vi "Default Instrument Setup.vi"(8 "error in (no error)":errorcluster, 11 "VISA resource name":refnum<visa-resource-name>) -> (0 "error out":errorcluster, 3 "VISA resource name out":refnum<visa-resource-name>)   [LabVIEW 2021, in "Keithley 24XX.lvlib"]
doc: "This Utility VI sends a default command string to the instrument whenever a new VISA session is opened, or the instrument is reset. Use this VI as a subVI for the Initialize and Reset VIs. Altering this VI could cause these two VIs to operate incorrectly."
uses:
  <instrlib>/Keithley 24XX/Keithley 24XX.lvlib
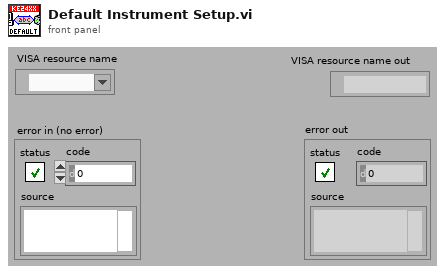
[diagram p1: front panel]
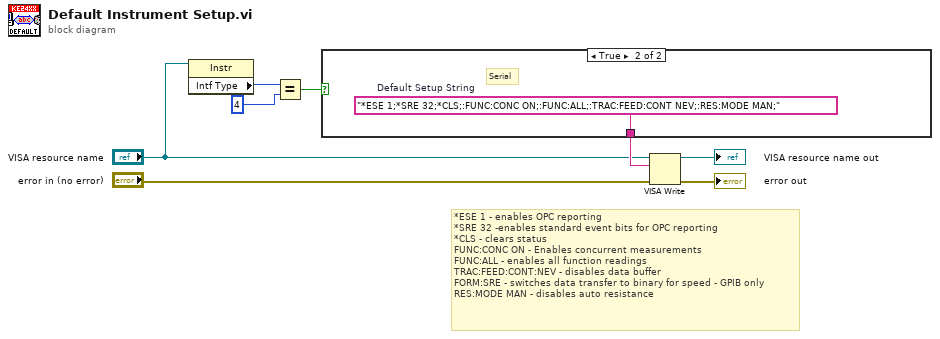
[diagram p0: block diagram]
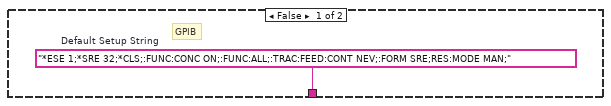
[diagram p2: hidden frame]
diagram:
  # "*ESE 1 - enables OPC reporting\n*SRE 32 -enables standard event bits for OPC reporting\n*CLS - clears status\nFUNC:CONC ON - Enables concurrent measurements\nFUNC:ALL - enables all function readings\nTRAC:FEED:CONT:NEV - disables data buffer\nFORM:SRE - switches data transfer to binary for speed - GPIB only\nRES:MODE MAN - disables auto resistance"
  n1 = property class="Instr"(reference="VISA resource name") -> ("Intf Type"=w2:u16)  [unwired: 1 in, 2 out]
  n2 = Equal?(x=w2, y=u16 4) -> (x = y?=w3:bool)
  n3 = case shown="True" w3 {
    tunnel: [w9 w10] -> w5
    frame False {
      w9 = "*ESE 1;*SRE 32;*CLS;:FUNC:CONC ON;:FUNC:ALL;:TRAC:FEED:CONT NEV;:FORM SRE;RES:MODE MAN;"  # Default Setup String
      # "GPIB"
    }
    frame True {
      w10 = "*ESE 1;*SRE 32;*CLS;:FUNC:CONC ON;:FUNC:ALL;:TRAC:FEED:CONT NEV;:RES:MODE MAN;"  # Default Setup String
      # "Serial"
    }
  }
  n4 = VISA Write(VISA resource name="VISA resource name", write buffer=w5, error in (no error)="error in (no error)") -> (VISA resource name out=→"VISA resource name out":refnum<visa-resource-name>, error out=→"error out":errorcluster)  [unwired: 1 out]
